vi "Pot Single Line.vi"() -> ()   [LabVIEW 2011]
uses:
  <vilib>/Utility/error.llb/DialogType.ctl
  Shared Components/Config Manager Class/Type Definitions/Named Position.ctl
  Shared Components/Gantry Class/Gantry Class.lvclass
  Shared Components/SyringeTool Class/SyringeTool Class.lvclass
  Shared Components/WorkTable Class/WorkTable Class.lvclass
  Shared Components/Config Manager Class/Type Definitions/Camera Enum.ctl
panel:
  in  "stop":bool
  in  "Pick Point":bool
  in  "Config Folder":path=path "C:/Users/Husker/Desktop/gantry/Config"
  out "preview":T1(plugin-control)
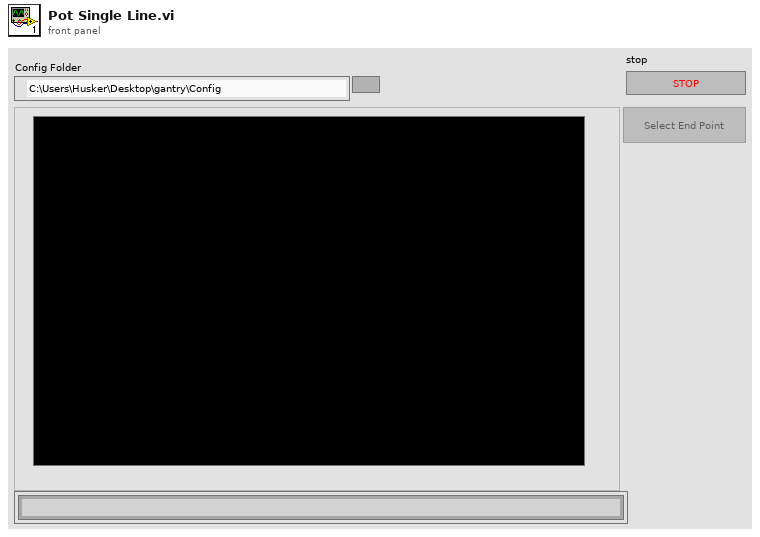
[diagram p1: front panel]
types:
  T1 = typedef "IMAQ Image.ctl" = refnum<image>
  T2 = typedef "Named Position.ctl" = enum16{"home", "module_chuck_0", "module_chuck_1", "module_chuck_2", "module_chuck_3", "module_chuck_4", "glue_reservoir_chuck", "stamp_tool_chuck", "weight_tool_chuck", "needle_calibration", "tool_rack_pos_0_in", "tool_rack_pos_0_out", "tool_rack_pos_1_in", "tool_rack_pos_1_out", "tool_rack_pos_2_in", "tool_rack_pos_2_out", "front_load_position"}
  T3 = typedef "DialogType.ctl" = u16
  T4 = enum8{"Enabled", "Disabled", "Disabled and Grayed Out"}
  T5 = typedef "Worktable_Syringe.ctl" = cluster{"Syringe Holder":enum16{"Empty", "Populated", "Calibrated"}, "Mixing Time":timestamp, "Tip Offset":refnum<class "Vec3d Class.lvclass">}
  T6 = typedef "Camera Enum.ctl" = enum16{"GANTRY HEAD", "NEEDLE CALIBRATION X", "NEEDLE CALIBRATION Y"}
  T7 = typedef "Physical Image.ctl" = cluster{"Image Position":refnum<class "Vec3d Class.lvclass">, "Image Reference":T1, "Field of View":cluster{"x(mm)":dbl, "y(mm)":dbl}}
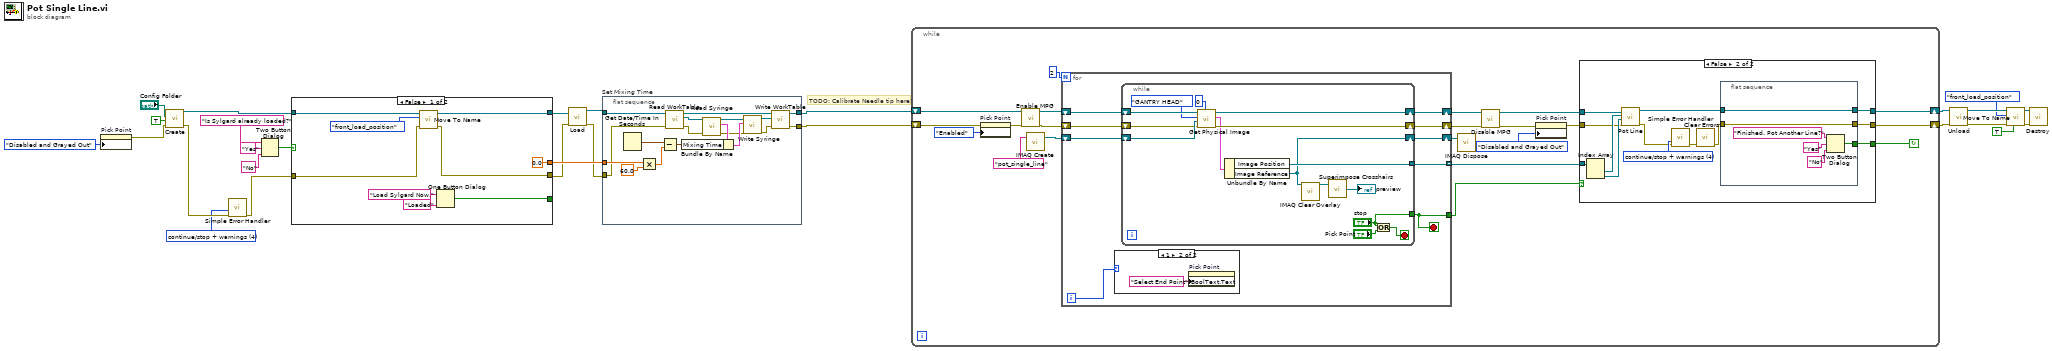
[diagram p0: block diagram]
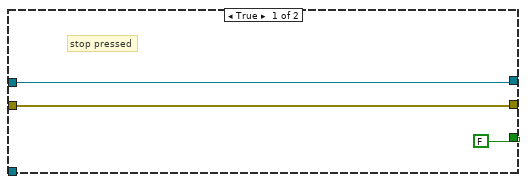
[diagram p2: hidden frame]
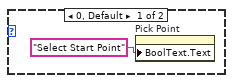
[diagram p3: hidden frame]
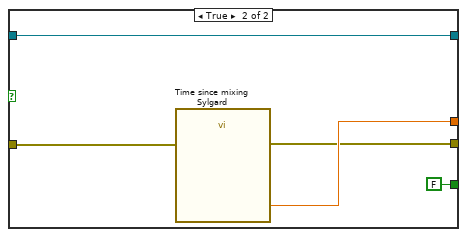
[diagram p4: hidden frame]
diagram:
  w5 = T3 4 items=["no dialog", "OK message", "continue or stop message", "OK message + warnings", "continue/stop + warnings"] ("type of dialog (OK msg:1)")
  # "TODO: Calibrate Needle tip here!"
  n1 = property on="Pick Point" class="Bool"("DisabledEnum"=T4."Disabled and Grayed Out" ("Disabled")) -> (error out=w8:errorcluster)  [unwired: 2 in, 1 out]
  n2 = call "Create.vi"("error in"=w8, "HOME?"=TRUE, "Config Folder"="Config Folder") -> ("error out"=w7:errorcluster, "Gantry out"=w26:refnum<class "Gantry Class.lvclass">)  [unwired: 7 in]
  n3 = call <vilib>:"Simple Error Handler.vi"("type of dialog (OK msg:1)"=w5, "error in (no error)"=w7) -> ("error out"=w6:errorcluster)  [unwired: 3 in, 4 out]
  n4 = Two Button Dialog(message="Is Sylgard already loaded?", 1:"No" ("F button name (\"Cancel\")"), 2:"Yes" ("T button name (\"OK\")")) -> (T button?=w21:bool)
  n5 = case shown="False" w21 {
    tunnel: w26 -> [w35 w37]
    tunnel: w6 -> [w34 w40]
    tunnel: [w32 w37] -> w20
    tunnel: [w31 w39] -> w18
    tunnel: [0.0 ("minutes") w41] -> w25
    tunnel: [w29 FALSE ("true")] -> _
    frame False {
      n6 = call-dynamic "Move To Name.vi"("error in"=w34, "Destination"=Named_Position."front_load_position", "Gantry in"=w35) -> ("error out"=w31:errorcluster, "Gantry out"=w32:refnum<class "Gantry Class.lvclass">)  [unwired: 7 in]
      n7 = One Button Dialog(message="Load Sylgard Now.", button name ("OK")="Loaded") -> (true=w29:bool)
    }
    frame True {
      n8 = call "Time since mixing Sylgard"("error in (no error)"=w40) -> ("minutes"=w41:dbl, "error out"=w39:errorcluster)  [unwired: 16 in, 1 out]
    }
  }
  n9 = call "Load.vi"("error in"=w18, "Gantry in"=w20) -> ("error out"=w17:errorcluster, "SyringeTool out"=w19:refnum<class "SyringeTool Class.lvclass">)  [unwired: 8 in]
  n10 = flat-sequence "Set Mixing Time" {
    tunnel: w19 -> [w55]
    tunnel: w25 -> [w59]
    tunnel: w17 -> [w54]
    tunnel: [w43] -> w3
    tunnel: [w42] -> w2
    frame #0 {
      n11 = Get Date/Time In Seconds() -> (seconds since 1Jan1904=w57:timestamp)
      n12 = Multiply(x=w59, y=60.0) -> (x*y=w56:dbl)
      n13 = Subtract(x=w57, y=w56) -> (x-y=w51:timestamp)
      n14 = call-dynamic "Read WorkTable.vi"("error in"=w54, "Gantry Class in"=w55) -> ("error out"=w46:errorcluster, "WorkTable Class.lvclass"=w53:refnum<class "WorkTable Class.lvclass">, "Gantry Class out"=w48:refnum<class "SyringeTool Class.lvclass">)  [unwired: 7 in]
      n15 = call "Read Syringe.vi"("error in"=w46, "WorkTable in"=w53) -> ("error out"=w45:errorcluster, "Syringe"=w52:T5, "WorkTable out"=w49:refnum<class "WorkTable Class.lvclass">)  [unwired: 7 in]
      n16 = Bundle By Name(cluster=w52, "Mixing Time"=w51) -> (w50:T5)
      n17 = call-dynamic "Write Syringe.vi"("error in (no error)"=w45, "Syringe"=w50, "WorkTable Class in"=w49) -> ("error out"=w44:errorcluster, "WorkTable Class out"=w47:refnum<class "WorkTable Class.lvclass">)  [unwired: 7 in]
      n18 = call-dynamic "Write WorkTable.vi"("error in (no error)"=w44, "WorkTable Class.lvclass"=w47, "Gantry Class in"=w48) -> ("error out"=w42:errorcluster, "Gantry Class out"=w43:refnum<class "SyringeTool Class.lvclass">)  [unwired: 7 in]
    }
  }
  n19 = while {
    shift-right: [w75] -> w16
    shift-left: w3 -> [w64]
    shift-right: [w74] -> w15
    shift-left: w2 -> [w72]
    stop <- w73 continue-if-true
    n20 = property on="Pick Point" class="Bool"(error in=w72, "DisabledEnum"=T4."Enabled" ("Disabled")) -> (error out=w62:errorcluster)  [unwired: 1 in, 1 out]
    n21 = call-dynamic "Enable MPG.vi"("error in"=w62, "Gantry in"=w64) -> ("error out"=w61:errorcluster, "Gantry out"=w63:refnum<class "SyringeTool Class.lvclass">)  [unwired: 8 in]
    n22 = call "IMAQ Create"("Image Name"="pot_single_line") -> ("New Image"=w78:T1)  [unwired: 4 in, 1 out]
    n23 = for {
      N: 2 -> [_]
      shift-right: [w108] -> w68
      shift-left: w63 -> [w110]
      shift-right: [w107] -> w77
      shift-left: w78 -> [w111]
      tunnel: [w106] -> w76 mode=indexing
      shift-right: [w105] -> w67
      shift-left: w61 -> [w109]
      tunnel: [w103] -> w60
      i -> [w104]
      stop <- w103 stop-if-true
      n24 = case shown="1" w104 {
        frame 0, Default {
          n25 = property on="Pick Point" class="Bool"("BoolText.Text"="Select Start Point" ("Boolean Text.Text")) -> ()  [unwired: 2 in, 2 out]
        }
        frame 1 {
          n26 = property on="Pick Point" class="Bool"("BoolText.Text"="Select End Point" ("Boolean Text.Text")) -> ()  [unwired: 2 in, 2 out]
        }
      }
      n27 = while {
        shift-right: [w125] -> w108
        shift-left: w110 -> [w127]
        tunnel: [w122] -> w106
        shift-right: [w120] -> w107
        shift-left: w111 -> [w128]
        shift-right: [w124] -> w105
        shift-left: w109 -> [w126]
        tunnel: ["stop"] -> w103
        stop <- w117 stop-if-true
        n28 = call-dynamic "Get Physical Image.vi"("Delay(milliseconds)"=0, "error in"=w126, "Image In"=w128, "Camera Name"=Camera_Enum."GANTRY HEAD", "Gantry in"=w127) -> ("error out"=w124:errorcluster, "Physical Image"=w123:T7, "Gantry out"=w125:refnum<class "SyringeTool Class.lvclass">)  [unwired: 4 in]
        n29 = Unbundle By Name(w123) -> ("Image Position"=w122:refnum<class "Vec3d Class.lvclass">, "Image Reference"=w120:T1)
        n30 = call "IMAQ Clear Overlay"("Image"=w120) -> ("Image Out"=w119:T1)  [unwired: 9 in, 1 out]
        n31 = call "Superimpose Crosshairs.vi"("Refnum in"=w119) -> ("Refnum out"=→"preview":T1)  [unwired: 1 in]
        n32 = Or(x="stop", y="Pick Point") -> (x .or. y?=w117:bool)
      }
    }
    n33 = call "IMAQ Dispose"("Image"=w77) -> ()  [unwired: 5 in, 1 out]
    n34 = call-dynamic "Disable MPG.vi"("error in"=w67, "Gantry in"=w68) -> ("error out"=w66:errorcluster, "Gantry out"=w65:refnum<class "SyringeTool Class.lvclass">)  [unwired: 8 in]
    n35 = property on="Pick Point" class="Bool"(error in=w66, "DisabledEnum"=T4."Disabled and Grayed Out" ("Disabled")) -> (error out=w70:errorcluster)  [unwired: 1 in, 1 out]
    n36 = case shown="False" w60 {
      tunnel: w76 -> [_ w96]
      tunnel: [w83 w90] -> w75
      tunnel: [w82 w88] -> w74
      tunnel: [FALSE ("T button?") w86] -> w73
      tunnel: w70 -> [w82 w85]
      tunnel: w65 -> [w83 w84]
      frame True {
        # "stop pressed"
      }
      frame False {
        w93 = T3 4 items=["no dialog", "OK message", "continue or stop message", "OK message + warnings", "continue/stop + warnings"] ("type of dialog (OK msg:1)")
        n37 = Index Array(array=w96) -> (element #1=w95:refnum<class "Vec3d Class.lvclass">, element #2=w94:refnum<class "Vec3d Class.lvclass">)  [unwired: 2 in]
        n38 = call-dynamic "Pot Line.vi"("error in"=w85, "End Position"=w94, "Start Position"=w95, "SyringeTool in"=w84) -> ("error out"=w92:errorcluster, "SyringeTool out"=w89:refnum<class "SyringeTool Class.lvclass">)  [unwired: 6 in]
        n39 = call <vilib>:"Simple Error Handler.vi"("type of dialog (OK msg:1)"=w93, "error in (no error)"=w92) -> ("error out"=w91:errorcluster)  [unwired: 3 in, 4 out]
        n40 = call <vilib>:"Clear Errors.vi"("error in (no error)"=w91) -> ("error out"=w87:errorcluster)  [unwired: 6 in]
        n41 = flat-sequence {
          tunnel: [w102] -> w90
          tunnel: w89 -> [w102]
          tunnel: [w101] -> w88
          tunnel: w87 -> [w101]
          tunnel: [w97] -> w86
          frame #0 {
            n42 = Two Button Dialog(message="Finished. Pot Another Line?", 1:"No" ("F button name (\"Cancel\")"), 2:"Yes" ("T button name (\"OK\")")) -> (T button?=w97:bool)
          }
        }
      }
    }
  }
  n43 = call "Unload.vi"("error in"=w15, "SyringeTool in"=w16) -> ("error out"=w14:errorcluster, "Gantry out"=w13:refnum<class "Gantry Class.lvclass">)  [unwired: 8 in]
  n44 = call-dynamic "Move To Name.vi"("Direct"=TRUE, "error in"=w14, "Destination"=Named_Position."front_load_position", "Gantry in"=w13) -> ("error out"=w12:errorcluster, "Gantry out"=w11:refnum<class "Gantry Class.lvclass">)  [unwired: 6 in]
  n45 = call "Destroy.vi"("error in"=w12, "Gantry Class in"=w11) -> ()  [unwired: 9 in, 1 out]
